vi "load standard into cycle.vi"(8 "error in":errorcluster) -> (0 "error out":errorcluster)   [LabVIEW 2016]
uses:
  controls/data control cluster.ctl
panel:
  out "output cluster":T1
  out "DATA CLUSTER in":T1
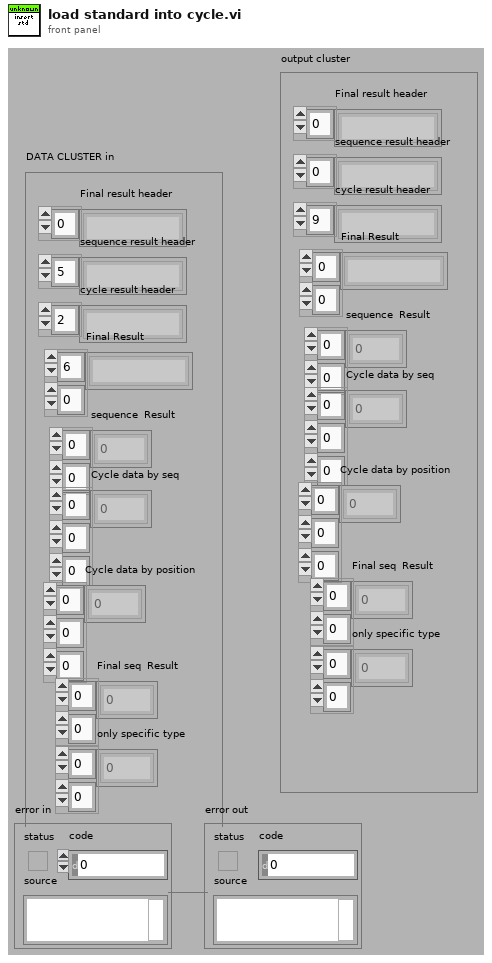
[diagram p1: front panel]
types:
  T1 = typedef "data control cluster.ctl" = cluster{"Final result header":string[], "sequence result header":string[], "cycle result header ":string[], "Final Result":string[][], "sequence  Result":dbl[][], "Cycle data by seq":dbl[][][], "Cycle data by position":dbl[][][], "Final seq  Result":dbl[][], "only specific type":dbl[][]}
  T2 = typedef "cycle results control.ctl" = cluster{"sample info":string[][], "cycle results labels":string[], "cycle results dbl":dbl[][]}
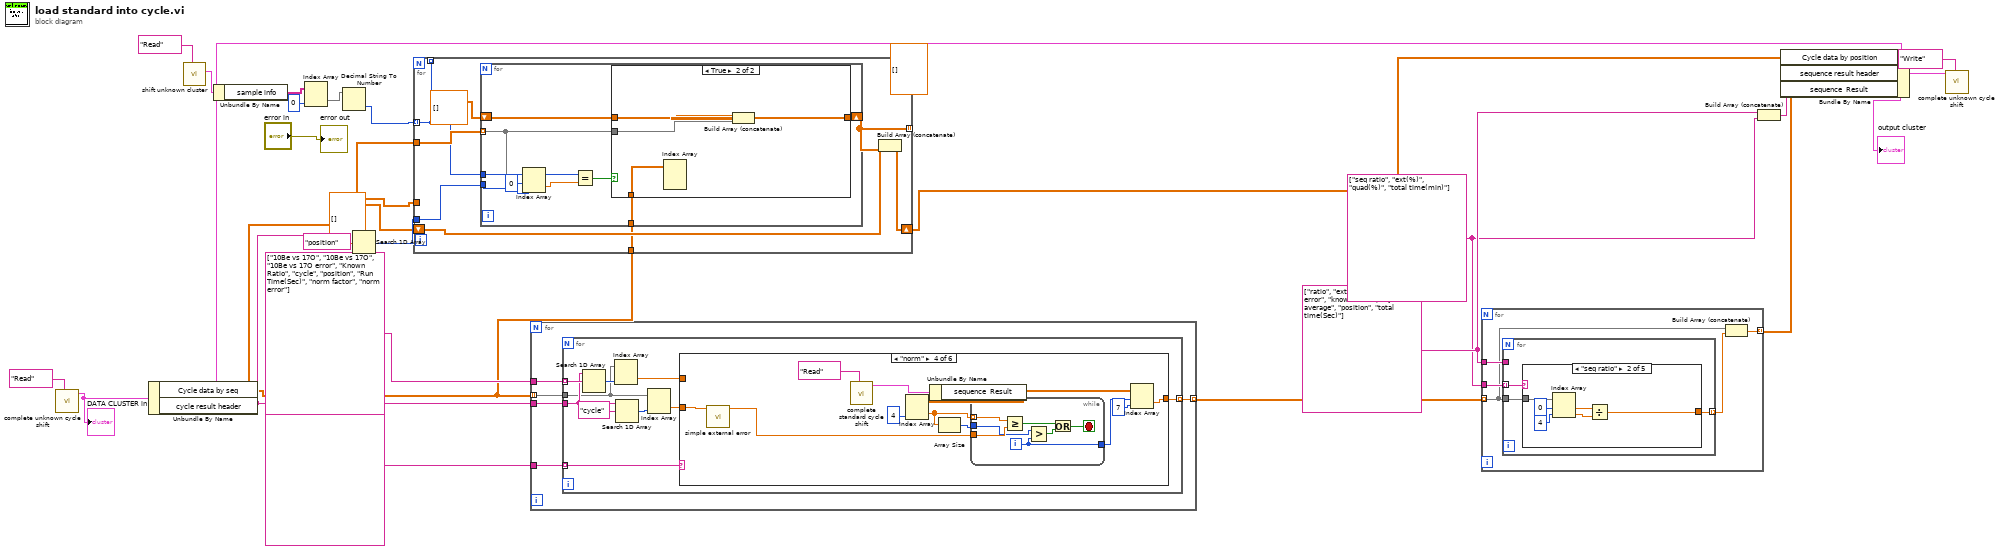
[diagram p0: block diagram]
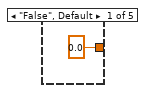
[diagram p3: hidden frame]
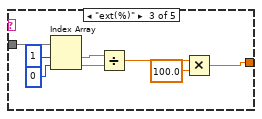
[diagram p4: hidden frame]
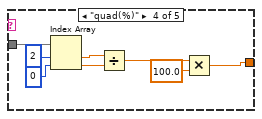
[diagram p5: hidden frame]
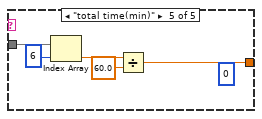
[diagram p6: hidden frame]
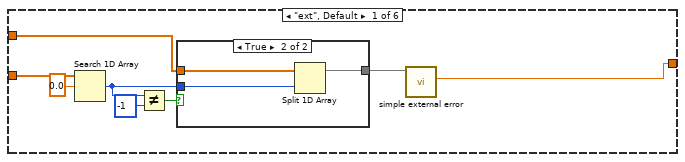
[diagram p7: hidden frame]
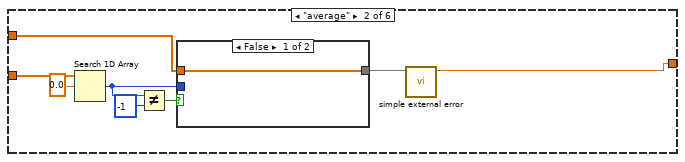
[diagram p9: hidden frame]
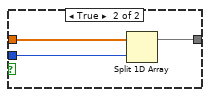
[diagram p10: hidden frame]
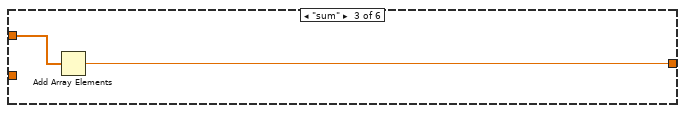
[diagram p11: hidden frame]
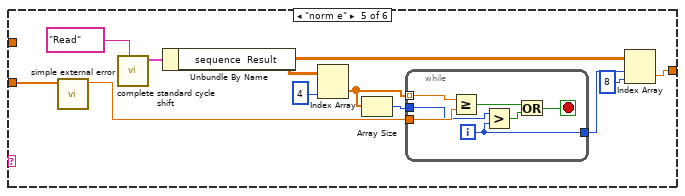
[diagram p12: hidden frame]
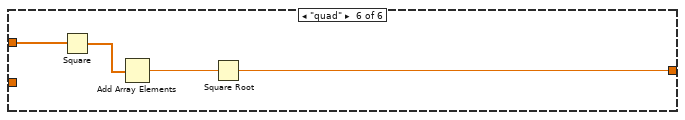
[diagram p13: hidden frame]
diagram:
  (unwired) dbl[][][] []
  w22 = string[] ["ratio", "ext error", "quad error", "known Ratio", "Cycle average", "position", "total time(Sec)"]
  w21 = string[] ["seq ratio", "ext(%)", "quad(%)", "total time(min)"]
  n1 = call "complete unknown cycle shift.vi"("read write shift"="Read") -> ("DATA CLUSTER out"=w18:T1)  [unwired: 9 in, 1 out]
  "DATA CLUSTER in" <- w18
  n2 = Unbundle By Name(w18) -> ("Cycle data by seq"=w2:dbl[][][], "cycle result header"=w16:string[])
  n3 = call "shift unknown cluster.vi"("read write shift"="Read") -> ("cycle results cluster out"=w9:T2)  [unwired: 9 in, 1 out]
  n4 = Unbundle By Name(w9) -> ("sample info"=w8:string[][])
  n5 = Index Array(array=w8, index (col)=0 ("disabled index (col)")) -> (element=w6:string[])  [unwired: 1 in]
  n6 = Decimal String To Number(string=w6) -> (number=w5:i32[])  [unwired: 2 in, 1 out]
  n7 = Search 1D Array(1D array=w16, element="position") -> (index of element=w11:i32)  [unwired: 1 in]
  n8 = for {
    tunnel: w2 -> [w32]
    tunnel: [w28] -> _ mode=indexing
    tunnel: w2 -> [_]
    tunnel: w11 -> [w30]
    tunnel: w5 -> [w26] mode=indexing
    shift-right: [w29] -> w1
    shift-left: dbl[][][] [] ("Cycle data by seq") -> [w27]
    tunnel: [w26] -> _ mode=indexing
    tunnel: w2 -> [w25]
    n9 = for {
      tunnel: w32 -> [w37] mode=indexing
      shift-right: [w39] -> w28
      shift-left: dbl[][] [] -> [w41]
      tunnel: w26 -> [w40]
      tunnel: w30 -> [w36]
      tunnel: w25 -> [w33]
      n10 = Index Array(array=w37, index (row)=0 ("disabled index (row)"), index (col)=w36) -> (element=w35:dbl)
      n11 = Equal?(x=w40, y=w35) -> (x = y?=w38:bool)
      n12 = case shown="True" w38 {
        tunnel: w37 -> [_ w46]
        tunnel: [w42 w45] -> w39
        tunnel: w41 -> [w42 w44]
        tunnel: w33 -> [_ w43]
        frame False {
        }
        frame True {
          n13 = Index Array(array=w43) -> ()  [unwired: 3 in, 1 out]
          n14 = Build Array (concatenate)(w44, w46) -> (w45:dbl[][])
        }
      }
    }
    n15 = Build Array (concatenate)(w27, w28) -> (w29:dbl[][][])
  }
  n16 = for {
    tunnel: w2 -> [w49] mode=indexing
    tunnel: w16 -> [w51]
    tunnel: string[] ["10Be vs 17O", "10Be vs 17O", "10Be vs 17O error", "Known Ratio", "cycle", "position", "Run Time(Sec)", "norm factor", "norm error"] -> [w50]
    tunnel: string[] ["average", "ext", "quad", "average", "average", "average", "sum", "norm", "norm e"] -> [w48]
    tunnel: [w47] -> w13 mode=indexing
    n17 = for {
      tunnel: w51 -> [w56]
      tunnel: w50 -> [w61] mode=indexing
      tunnel: w49 -> [w54]
      tunnel: w48 -> [w60] mode=indexing
      tunnel: [w58] -> w47 mode=indexing
      n18 = Search 1D Array(1D array=w56, element=w61) -> (index of element=w57:i32)  [unwired: 1 in]
      n19 = Index Array(array=w54, index (col)=w57) -> (element=w59:dbl[])  [unwired: 1 in]
      n20 = Search 1D Array(1D array=w56, element="cycle") -> (index of element=w53:i32)  [unwired: 1 in]
      n21 = Index Array(array=w54, index (col)=w53) -> (element=w52:dbl[])  [unwired: 1 in]
      n22 = case shown="\"norm\"" w60 {
        tunnel: w59 -> [w67 w79 w87 _ _ w127]
        tunnel: [w69 w81 w86 w89 w107 w124] -> w58
        tunnel: w52 -> [w62 w74 _ w96 w114 _]
        frame "ext", Default {
          n23 = Search 1D Array(1D array=w62, element=0.0) -> (index of element=w64:i32)  [unwired: 1 in]
          n24 = Not Equal?(x=w64, y=-1) -> (x != y?=w65:bool)
          n25 = case shown="True" w65 {
            tunnel: w64 -> [_ w73]
            tunnel: w67 -> [w70 w72]
            tunnel: [w70 w71] -> w66
            frame False {
            }
            frame True {
              n26 = Split 1D Array(array=w72, index=w73) -> (first subarray=w71:dbl[])  [unwired: 1 out]
            }
          }
          n27 = call "simple external error.vi"("cycle results"=w66) -> ("External error"=w69:dbl)  [unwired: 7 in, 3 out]
        }
        frame "average" {
          n28 = Search 1D Array(1D array=w74, element=0.0) -> (index of element=w76:i32)  [unwired: 1 in]
          n29 = Not Equal?(x=w76, y=-1) -> (x != y?=w77:bool)
          n30 = case shown="False" w77 {
            tunnel: w76 -> [_ w85]
            tunnel: w79 -> [w82 w84]
            tunnel: [w82 w83] -> w78
            frame False {
            }
            frame True {
              n31 = Split 1D Array(array=w84, index=w85) -> (first subarray=w83:dbl[])  [unwired: 1 out]
            }
          }
          n32 = call "simple external error.vi"("cycle results"=w78) -> ("Sequence result"=w81:dbl)  [unwired: 7 in, 3 out]
        }
        frame "sum" {
          n33 = Add Array Elements(numeric array=w87) -> (sum=w86:dbl)
        }
        frame "norm" {
          n34 = call "simple external error.vi"("cycle results"=w96) -> ("Sequence result"=w95:dbl)  [unwired: 7 in, 3 out]
          n35 = call "complete standard cycle shift.vi"("read write shift"="Read") -> ("DATA CLUSTER out"=w97:T1)  [unwired: 9 in, 1 out]
          n36 = Unbundle By Name(w97) -> ("sequence  Result"=w88:dbl[][])
          n37 = Index Array(array=w88, index (col)=4 ("disabled index (col)")) -> (element=w93:dbl[])  [unwired: 1 in]
          n38 = Array Size(array=w93) -> (size(s)=w92:i32)
          n39 = while {
            tunnel: w95 -> [w104]
            tunnel: w93 -> [w105] mode=indexing
            tunnel: w92 -> [w103]
            tunnel: [w99] -> w91
            i -> [w99]
            stop <- w100 stop-if-true
            n40 = Greater Or Equal?(x=w105, y=w104) -> (x >= y?=w102:bool)
            n41 = Greater?(x=w103, y=w99) -> (0:w101:bool)
            n42 = Or(x=w102, y=w101) -> (x .or. y?=w100:bool)
          }
          n43 = Index Array(array=w88, index (row)=w91, index (col)=7) -> (element=w89:dbl)
        }
        frame "norm e" {
          n44 = call "simple external error.vi"("cycle results"=w114) -> ("Sequence result"=w113:dbl)  [unwired: 7 in, 3 out]
          n45 = call "complete standard cycle shift.vi"("read write shift"="Read") -> ("DATA CLUSTER out"=w115:T1)  [unwired: 9 in, 1 out]
          n46 = Unbundle By Name(w115) -> ("sequence  Result"=w106:dbl[][])
          n47 = Index Array(array=w106, index (col)=4 ("disabled index (col)")) -> (element=w111:dbl[])  [unwired: 1 in]
          n48 = Array Size(array=w111) -> (size(s)=w110:i32)
          n49 = while {
            tunnel: w113 -> [w122]
            tunnel: w111 -> [w123] mode=indexing
            tunnel: w110 -> [w121]
            tunnel: [w117] -> w109
            i -> [w117]
            stop <- w118 stop-if-true
            n50 = Greater Or Equal?(x=w123, y=w122) -> (x >= y?=w120:bool)
            n51 = Greater?(x=w121, y=w117) -> (0:w119:bool)
            n52 = Or(x=w120, y=w119) -> (x .or. y?=w118:bool)
          }
          n53 = Index Array(array=w106, index (row)=w109, index (col)=8) -> (element=w107:dbl)
        }
        frame "quad" {
          n54 = Square(x=w127) -> (x^2=w126:dbl[])
          n55 = Add Array Elements(numeric array=w126) -> (sum=w125:dbl)
          n56 = Square Root(x=w125) -> (sqrt(x)=w124:dbl)
        }
      }
    }
  }
  n57 = for {
    tunnel: w13 -> [w129] mode=indexing
    tunnel: w21 -> [w132]
    tunnel: w22 -> [w131]
    tunnel: [w128] -> w3 mode=indexing
    n58 = for {
      tunnel: w132 -> [w135] mode=indexing
      tunnel: w131 -> [_]
      tunnel: w129 -> [w134]
      tunnel: [w133] -> w130 mode=indexing
      n59 = case shown="\"seq ratio\"" w135 {
        tunnel: w134 -> [_ w142 w150 w158 w163]
        tunnel: [0.0 w137 w143 w151 w159] -> w133
        frame "False", Default {
        }
        frame "seq ratio" {
          n60 = Index Array(array=w142, index #1=0 ("index"), index #2=4 ("index")) -> (element #1=w138:dbl, element #2=w139:dbl)
          n61 = Divide(x=w138, y=w139) -> (x/y=w137:dbl)
        }
        frame "ext(%)" {
          n62 = Index Array(array=w150, index #1=1 ("index"), index #2=0 ("index")) -> (element #1=w146:dbl, element #2=w147:dbl)
          n63 = Divide(x=w146, y=w147) -> (x/y=w145:dbl)
          n64 = Multiply(x=w145, y=100.0) -> (x*y=w143:dbl)
        }
        frame "quad(%)" {
          n65 = Index Array(array=w158, index #1=2 ("index"), index #2=0 ("index")) -> (element #1=w154:dbl, element #2=w155:dbl)
          n66 = Divide(x=w154, y=w155) -> (x/y=w153:dbl)
          n67 = Multiply(x=w153, y=100.0) -> (x*y=w151:dbl)
        }
        frame "total time(min)" {
          (unwired) 0 ("index")
          n68 = Index Array(array=w163, index=6) -> (element=w161:dbl)
          n69 = Divide(x=w161, y=60.0) -> (x/y=w159:dbl)
        }
      }
    }
    n70 = Build Array (concatenate)(w129, w130) -> (w128:dbl[])
  }
  n71 = Build Array (concatenate)(w22, w21) -> (w20:string[])
  n72 = Bundle By Name(cluster=w18, "Cycle data by position"=w1, "sequence result header"=w20, "sequence  Result"=w3) -> (w14:T1)
  "output cluster" <- w14
  n73 = call "complete unknown cycle shift.vi"("read write shift"="Write", "DATA CLUSTER in"=w14) -> ()  [unwired: 8 in, 2 out]
  "error out" <- "error in"
